vi "read_PulseDelay.vi"() -> ()   [LabVIEW 2014]
panel:
  out "PulseDelay":dbl
  in  "Num Bytes to Fetch (64)":u8=64 min=1
  in  "Address (0x50)":u16=80 max=1023 format="%.0x"
  in  "Aardvark Handle":i32 min=0
  out "error out":errorcluster
  in  "error in (no error)":errorcluster
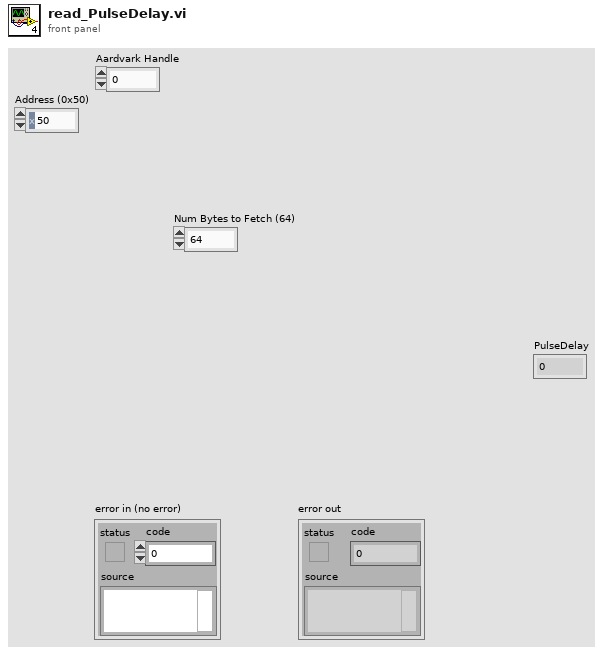
[diagram p1: front panel]
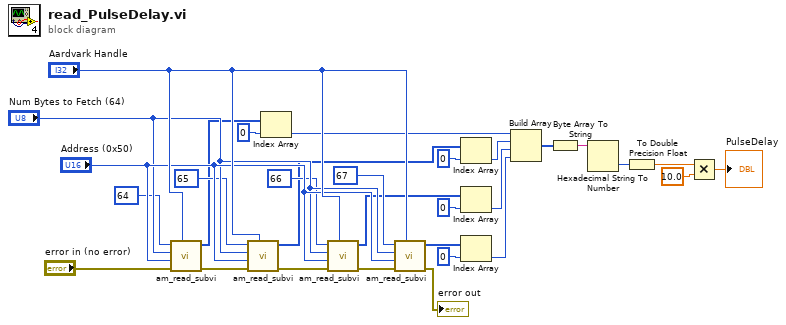
[diagram p0: block diagram]
diagram:
  n1 = call "am_read_subvi.vi"("Aardvark Handle in"="Aardvark Handle", "error in (no error)"="error in (no error)", "Address (0x50) in"="Address (0x50)", "Num Bytes to Fetch (64)"="Num Bytes to Fetch (64)", "Memory ADD"=u16 64) -> ("error out"=w29:errorcluster, "Array"=w17:u8[])  [unwired: 5 in]
  n2 = call "am_read_subvi.vi"("Aardvark Handle in"="Aardvark Handle", "error in (no error)"=w29, "Address (0x50) in"="Address (0x50)", "Num Bytes to Fetch (64)"="Num Bytes to Fetch (64)", "Memory ADD"=u16 65) -> ("error out"=w28:errorcluster, "Array"=w13:u8[])  [unwired: 5 in]
  n3 = Index Array(array=w17, index=0) -> (element=w10:u8)
  n4 = call "am_read_subvi.vi"("Aardvark Handle in"="Aardvark Handle", "error in (no error)"=w28, "Address (0x50) in"="Address (0x50)", "Num Bytes to Fetch (64)"="Num Bytes to Fetch (64)", "Memory ADD"=u16 66) -> ("error out"=w27:errorcluster, "Array"=w12:u8[])  [unwired: 5 in]
  n5 = call "am_read_subvi.vi"("Aardvark Handle in"="Aardvark Handle", "error in (no error)"=w27, "Address (0x50) in"="Address (0x50)", "Num Bytes to Fetch (64)"="Num Bytes to Fetch (64)", "Memory ADD"=u16 67) -> ("error out"=→"error out":errorcluster, "Array"=w11:u8[])  [unwired: 5 in]
  n6 = Index Array(array=w13, index=0) -> (element=w9:u8)
  n7 = Index Array(array=w12, index=0) -> (element=w8:u8)
  n8 = Index Array(array=w11, index=0) -> (element=w7:u8)
  n9 = Build Array(w10, w9, w8, w7) -> (w5:u8[])
  n10 = Byte Array To String(unsigned byte array=w5) -> (string=w4:string)
  n11 = Hexadecimal String To Number(string=w4) -> (number=w2:u32)  [unwired: 2 in, 1 out]
  n12 = To Double Precision Float(number=w2) -> (double precision float=w1:dbl)
  n13 = Multiply(x=w1, y=10.0) -> (x*y=→"PulseDelay":dbl)
